vi "FPGA_convert_pannel-channel-to-U16-Merlin.vi"(1 "pannel|channel":u16) -> (0 "Numérique":u16)   [LabVIEW 2013]
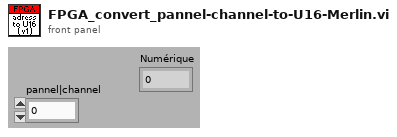
[diagram p1: front panel]
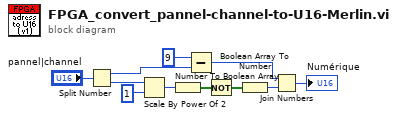
[diagram p0: block diagram]
diagram:
  n1 = Split Number(x="pannel|channel") -> (hi(x)=w2:u8, lo(x)=w5:u8)
  n2 = Scale By Power Of 2(n=w5, x=u8 1) -> (x*2^n=w9:u8)
  n3 = Number To Boolean Array(number=w9) -> (Boolean array=w10:bool[])
  n4 = Subtract(x=u8 9, y=w2) -> (x-y=w3:u8)
  n5 = Not(x=w10) -> (.not. x?=w11:bool[])
  n6 = Boolean Array To Number(Boolean array=w11) -> (number=w4:u8)
  n7 = Join Numbers(hi=w3, lo=w4) -> ((hi.lo)=→"Numérique":u16)
